vi "STAGE+mono+counter_edit11.vi"() -> ()   [LabVIEW 2017]
uses:
  Control 1.ctl
panel:
  out "XY Graph":cluster{dbl[], dbl[]}(graph)
  out "Slide":u8(slide) max=10 step=10 scale=0.0..10.0
  out "?":cluster{dbl[], "Y":T1}(graph)
  in  "?":enum32{"DELAY", "COUNTER", "MONO", "PLOT"}(tab)
  out "Final time [ps]":dbl
  out "Current time [ps]":dbl
  out "Initial time [ps]":dbl
  in  "Set this as t0":bool
  in  "Axis":i32=1
  in  "Motor ON":bool
  in  "Motor OFF":bool
  out "Current Position [mm]":dbl
  out "Final Position [mm]":dbl
  in  "Data Points":i32=100
  out "Current Point":i32
  in  "Step Size [um]":i32=10
  in  "Target [mm]":dbl format="%.3f"
  in  "Move":bool
  out "Initial position [mm]":dbl
  in  "GPIB address":string="23"
  in  "Count Mode":u16(ring) items=["A,B for Preset T", "A-B for Preset T", "A+B for Preset T", "A for Preset B"]
  in  "Trigger mode":u16(ring) items=["10 MHz"=0, "Input 2"=2, "Input T"=3]
  in  "Channel A Input":u16(ring)=1 items=["10 MHz", "Input 1"]
  in  "Channel B Input":u16(ring)=2 items=["Input 1"=1, "Input 2"=2]
  in  "Number of Measurements\n to take at one point/ Number of Periods":u16=1 min=1 max=2000 step=1
  in  "Time between measurements\n at one point (s)/Dwell Time":dbl=0.002 min=0.002 max=60.0 step=0.001
  in  "gate A mode (CW:0)":i16(slide) scale=0.0..2.0 scale format="%.2f"
  out "Counts":i32
  in  "Integrating time, 10^-7 sec":dbl=10000000.0
  out "Mono port":T2(ring)
  out "Time delay":u32=450000 min=1
  out "Serial":u32=12345
  in  "Step size":dbl=10.0 min=0.0
  in  "Scan to":i32=4000
  in  "Scan from":i32=2600
  out "Current wavelength":dbl
  out "Grt#":u8=1 min=1 max=3 step=1
  in  "?":bool
  out "Groove/mm":u32=1200
  out "Blaze (nm)":u32=300
  in  "Numeric 11":dbl
  in  "Numeric 10":dbl
  in  "Numeric 9":dbl
  in  "Numeric 8":dbl
  in  "Numeric 7":dbl
  in  "Numeric 6":dbl
  in  "Numeric 5":dbl
  in  "Numeric 4":dbl
  in  "Numeric 3":dbl
  in  "Numeric 2":dbl
  in  "Numeric":dbl
  out "Timeout 2":bool
  in  "?":bool
  out "Timeout":bool
  in  "Collect Data!":bool
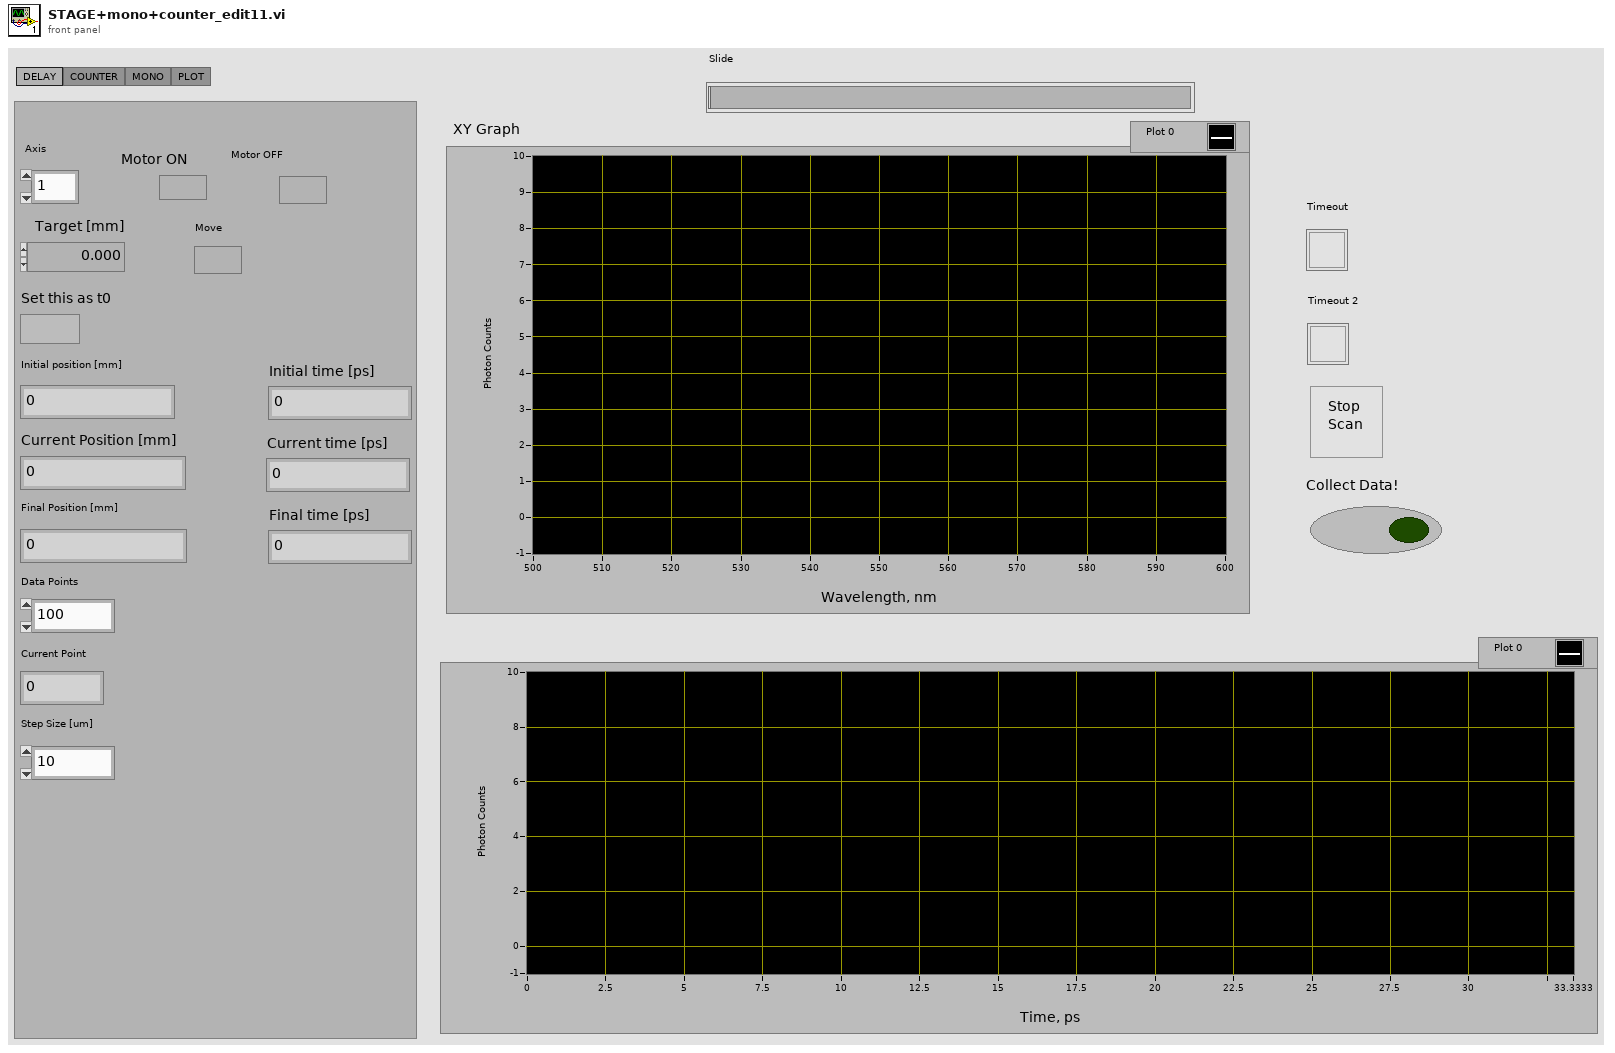
[diagram p1: front panel]
types:
  T1 = typedef "Control 1.ctl" = dbl[]
  T2 = enum8{"COM 1", "COM 2", "COM 3", "COM 4", "COM 5", "COM 6", "COM 7", "COM 8", "COM 9"}
  T3 = cluster{"input XON/XOFF":bool, "input HW Handshake":bool, "input alt HW HShk":bool, "output XON/XOFF":bool, "output HW Handshake":bool, "output alt HW HShk":bool, "XOFF byte":u8, "XON byte":u8, "parity error byte":u16}
  T4 = enum16{"no parity", "odd parity", "even parity", "mark parity", "space parity"}
  T5 = cluster{"Y[0]":dbl, "Y[1]":dbl, "Y[2]":dbl, "Y[3]":dbl, "Y[4]":dbl, "Y[5]":dbl, "Y[6]":dbl, "Y[7]":dbl, "Y[8]":dbl}
  T6 = typedef "NI_Matrix.lvlib/RealMatrix.ctl" = dbl[][]
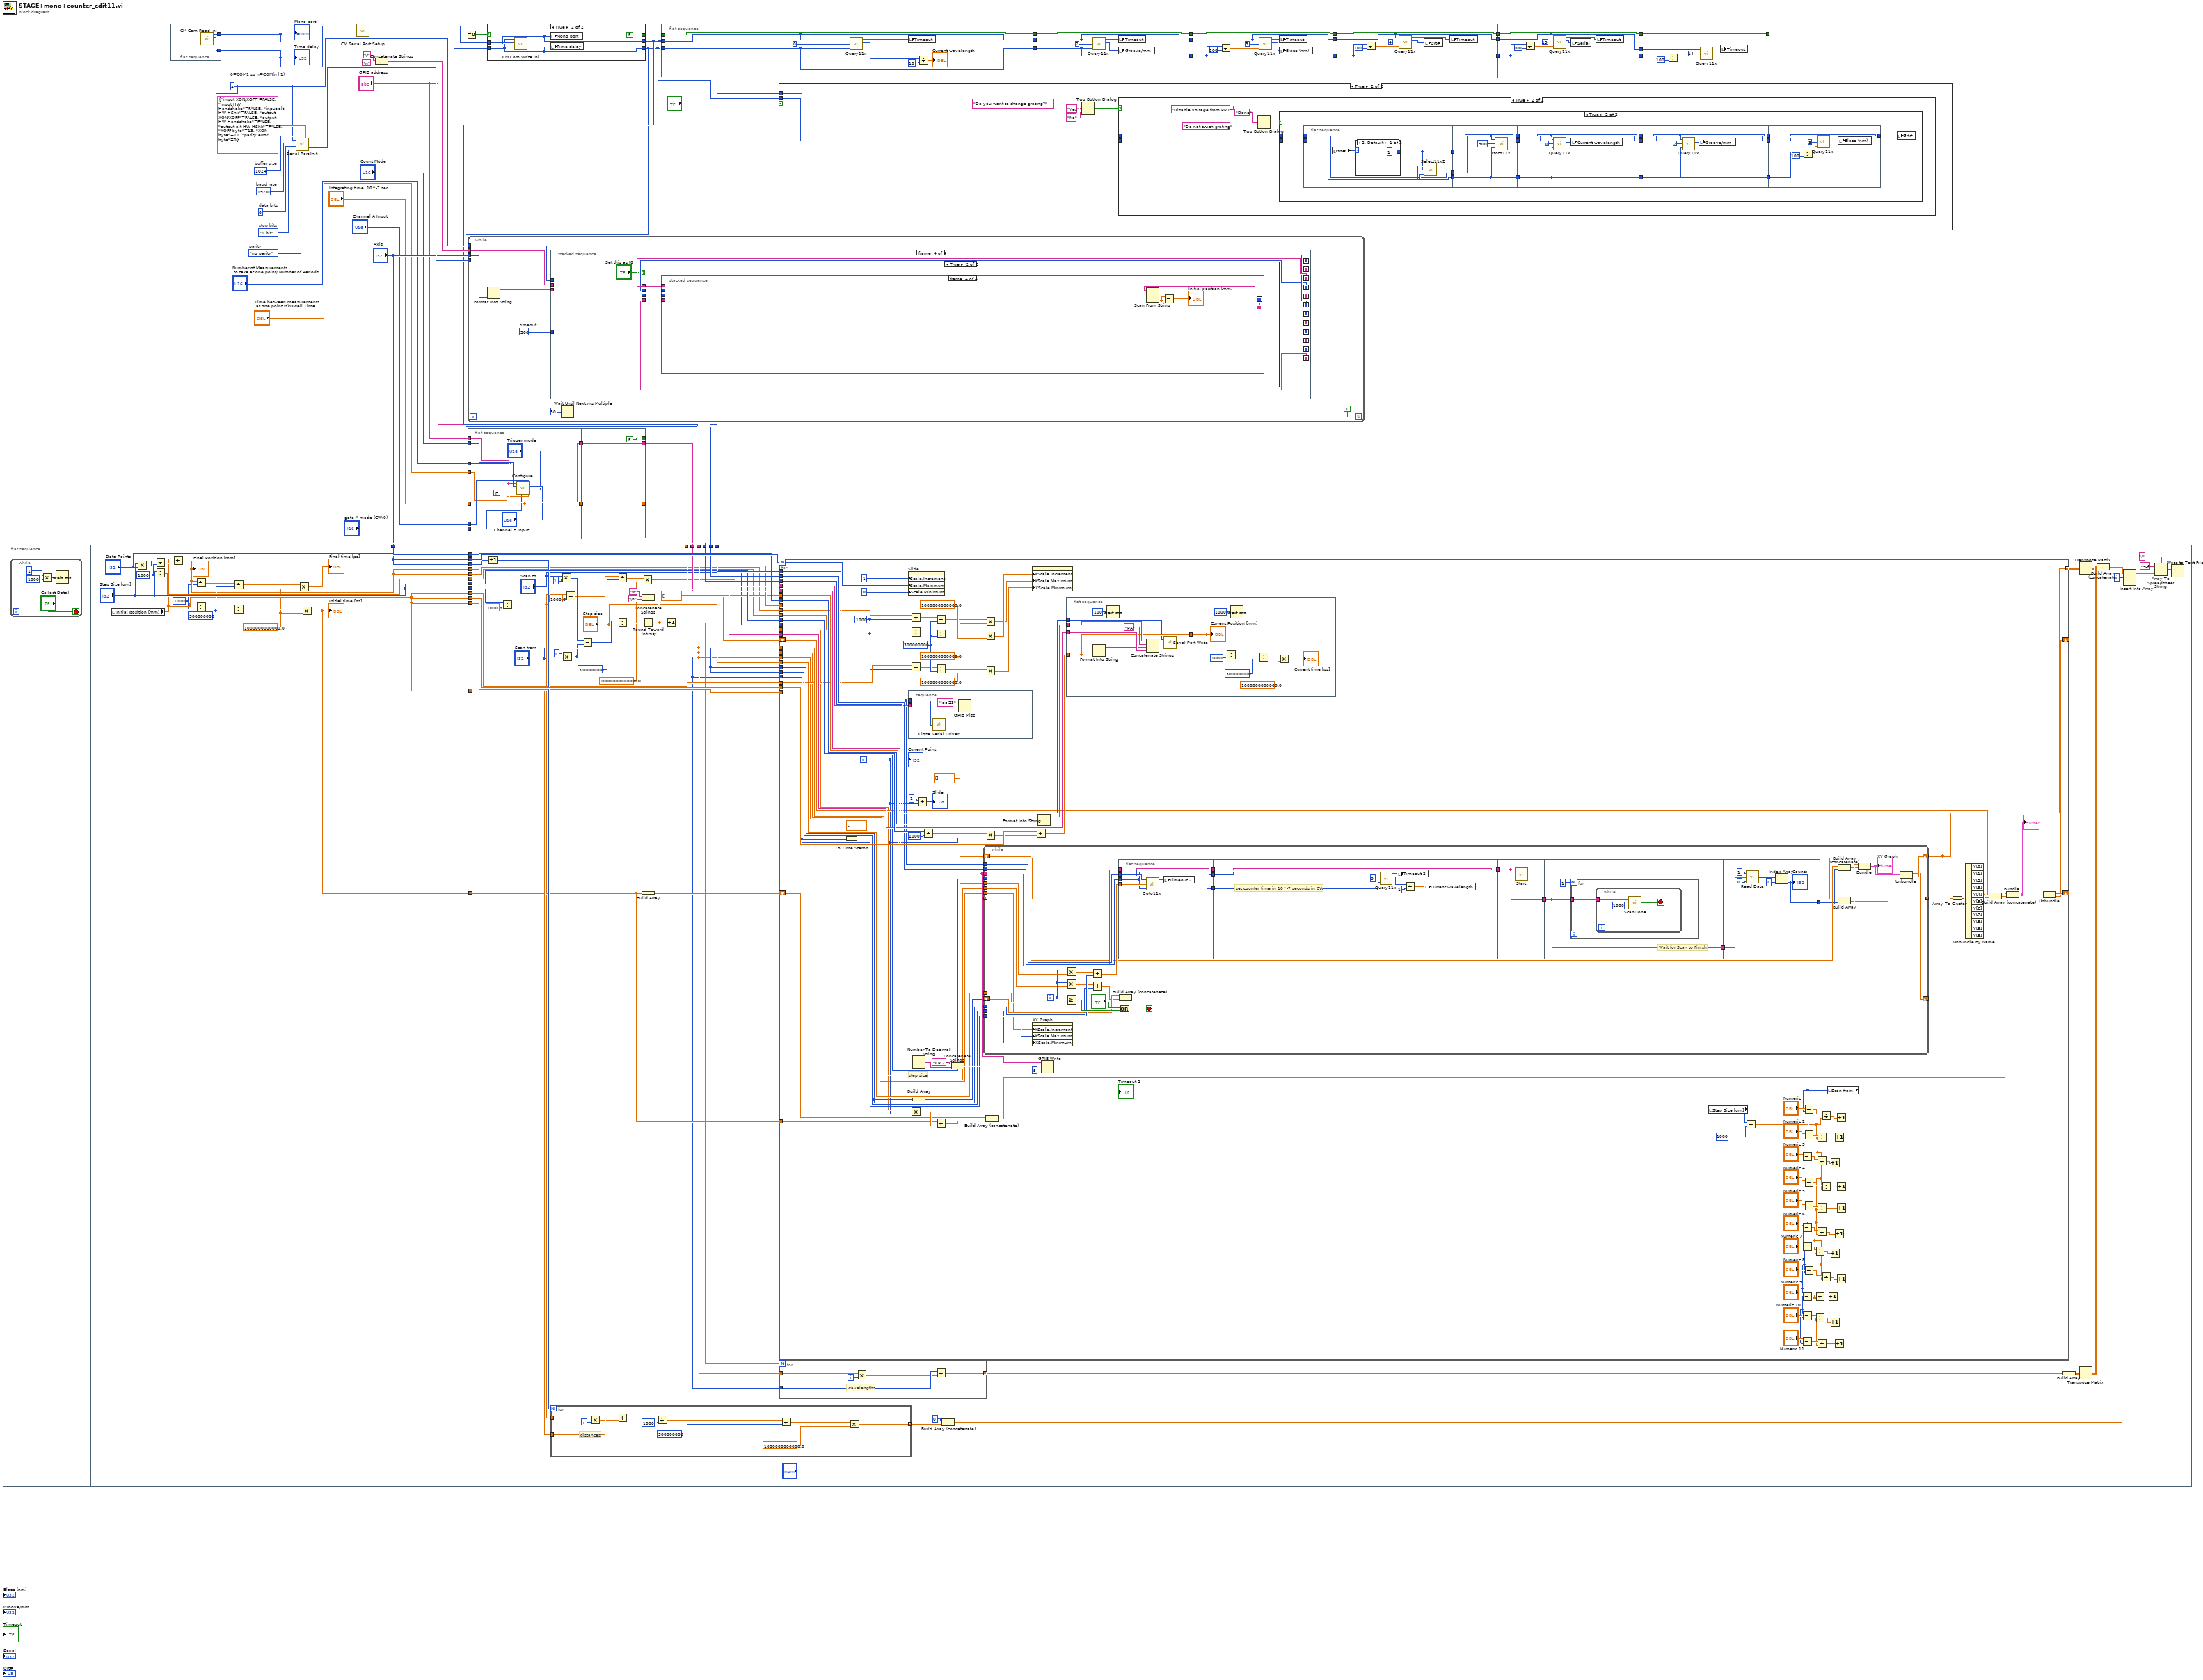
[diagram p0: block diagram]
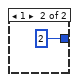
[diagram p5: hidden frame]
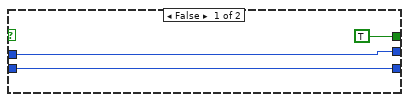
[diagram p6: hidden frame]
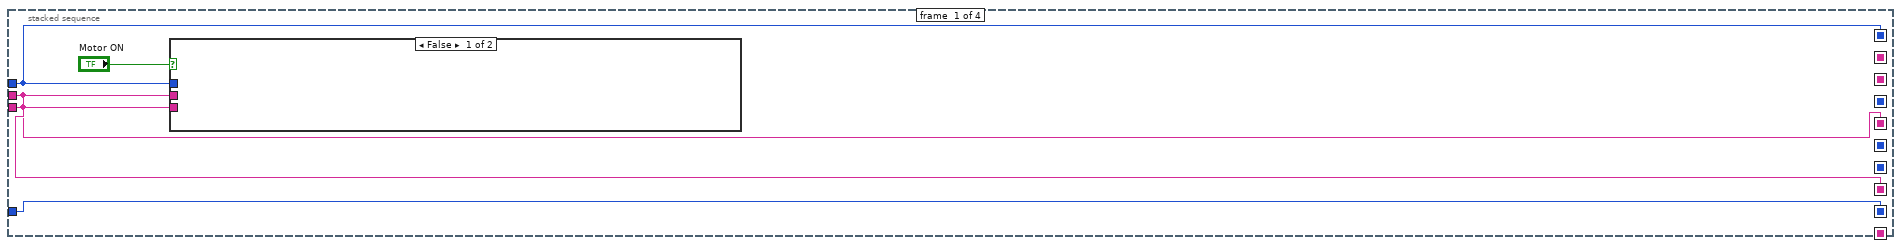
[diagram p7: hidden frame]
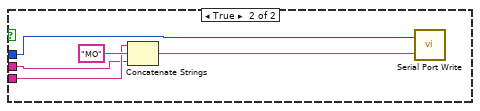
[diagram p8: hidden frame]
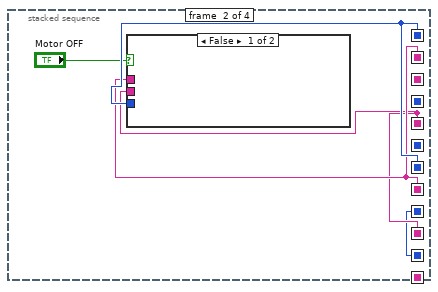
[diagram p9: hidden frame]
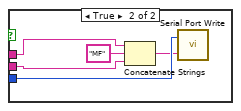
[diagram p10: hidden frame]
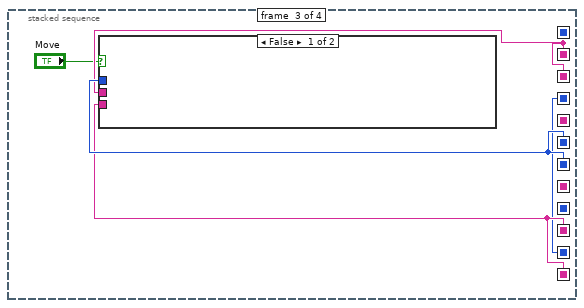
[diagram p11: hidden frame]
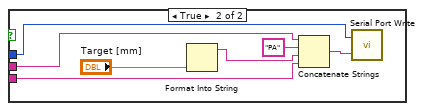
[diagram p12: hidden frame]
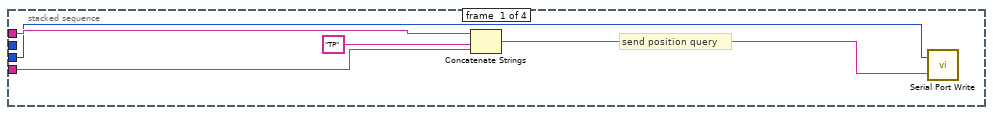
[diagram p14: hidden frame]
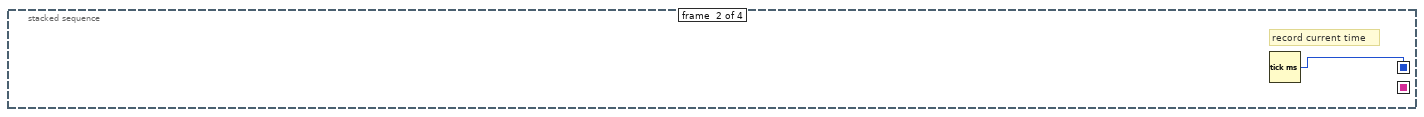
[diagram p15: hidden frame]
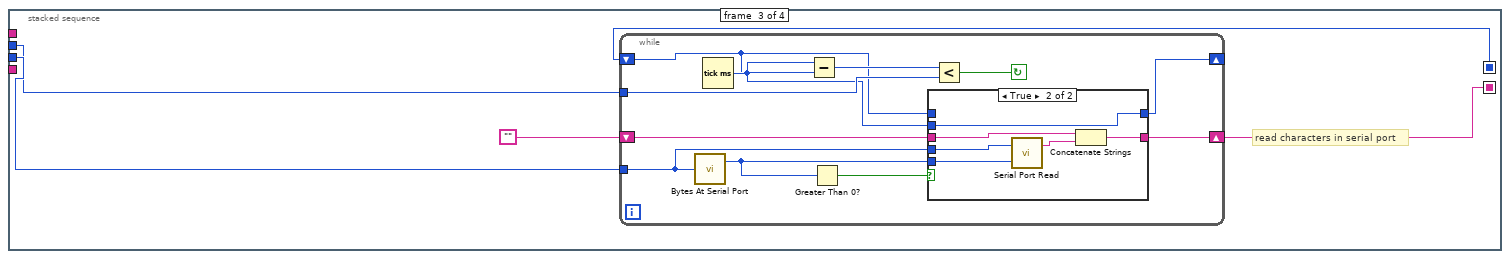
[diagram p16: hidden frame]
diagram:
  w55 = u32 19200  # baud rate
  w54 = u16 8  # data bits
  w53 = enum16{"1 bit", "1.5 bits", "2 bits"}."1 bit"  # stop bits
  w57 = T4."no parity"  # parity
  w52 = 4  # 0=COM1 so n=COM(n+1)
  w56 = u16 1024  # buffer size
  n1 = flat-sequence {
    tunnel: ["Data Points"] -> w61
    tunnel: "Axis" -> [w83]
    tunnel: [w75] -> w60
    tunnel: [w83] -> w59
    tunnel: ["Step Size [um]"] -> w12
    tunnel: [w75] -> w11
    tunnel: ["Step Size [um]"] -> w10
    tunnel: ["Data Points"] -> w9
    tunnel: [w75] -> w8
    tunnel: [w74] -> w7
    tunnel: [w75] -> w4
    tunnel: [w74] -> w3
    tunnel: [w77] -> w2
    tunnel: [w66] -> w1
    tunnel: w61 -> [w141]
    tunnel: w60 -> [w140]
    tunnel: w59 -> [w139]
    tunnel: w52 -> [w135]
    tunnel: w16 -> [w134]
    tunnel: w15 -> [w133]
    tunnel: w14 -> [w132]
    tunnel: "GPIB address" -> [w131]
    tunnel: w12 -> [w116]
    tunnel: w11 -> [w114]
    tunnel: w10 -> [w113]
    tunnel: w9 -> [w111]
    tunnel: w8 -> [w104]
    tunnel: w7 -> [w103]
    tunnel: w6 -> [w102]
    tunnel: w4 -> [w100]
    tunnel: w3 -> [w99]
    tunnel: w2 -> [w98]
    tunnel: w1 -> [w94]
    frame #0 {
      n2 = while {
        stop <- "Collect Data!" stop-if-true
        n3 = Multiply(x=1, y=1000) -> (x*y=w65:i32)
        n4 = Wait (ms)(milliseconds to wait=w65) -> ()  [unwired: 1 out]
      }
    }
    frame #1 {
      w67 = 1000000000000.0
      w73 = 1000
      w76 = 300000000
      w78 = 1000
      n5 = local read "Initial position [mm]"() -> (w75:dbl)
      n6 = Multiply(x="Step Size [um]", y="Data Points") -> (x*y=w82:i32)
      n7 = Divide(x=w82, y=w78) -> (x/y=w81:dbl)
      n8 = Divide(x="Step Size [um]", y=w78) -> (x/y=w77:dbl)
      n9 = Add(x=w75, y=w81) -> (x+y=w74:dbl)
      "Final Position [mm]" <- w74
      n10 = Divide(x=w74, y=w73) -> (x/y=w72:dbl)
      n11 = Divide(x=w75, y=w73) -> (x/y=w71:dbl)
      n12 = Divide(x=w72, y=w76) -> (x/y=w69:dbl)
      n13 = Divide(x=w71, y=w76) -> (x/y=w70:dbl)
      n14 = Multiply(x=w69, y=w67) -> (x*y=→"Final time [ps]":dbl)
      n15 = Multiply(x=w70, y=w67) -> (x*y=w66:dbl)
      "Initial time [ps]" <- w66
    }
    frame #2 {
      n16 = Increment(x=w111) -> (x+1=w112:i32)
      n17 = Divide(x=w116, y=1000.0) -> (x/y=w88:dbl)
      n18 = for {
        N: w112 -> [_]
        tunnel: w88 -> [w152]
        tunnel: w114 -> [w150]
        tunnel: [w143] -> w110 mode=indexing
        i -> [w151]
        # "distances"
        n19 = Multiply(x=w152, y=w151) -> (x*y=w149:dbl)
        n20 = Add(x=w150, y=w149) -> (x+y=w148:dbl)
        n21 = Divide(x=w148, y=1000) -> (x/y=w142:dbl)
        n22 = Divide(x=w142, y=300000000) -> (x/y=w145:dbl)
        n23 = Multiply(x=w145, y=1000000000000.0) -> (x*y=w143:dbl)
      }
      n24 = Multiply(x="Scan to", y=1) -> (x*y=w95:i32)
      n25 = Multiply(x=1, y="Scan from") -> (x*y=w84:i32)
      n26 = Divide(x=w88, y=1000.0) -> (x/y=w89:dbl)
      n27 = Subtract(x=w95, y=w84) -> (x-y=w126:i32)
      n28 = Divide(x=w89, y=300000000) -> (x/y=w91:dbl)
      n29 = Divide(x=w126, y="Step size") -> (x/y=w125:dbl)
      n30 = Multiply(x=w91, y=1000000000000.0) -> (x*y=w87:dbl)
      n31 = Concatenate Strings("\r", "\n") -> (w136:string)
      n32 = Round Toward -Infinity(1:w125) -> (0:w124:dbl)
      n33 = Build Array(w94) -> (w96:dbl[])
      n34 = Increment(x=w124) -> (x+1=w123:dbl)
      n35 = for {
        N: w141 -> [w226]
        tunnel: w140 -> [w262]
        tunnel: w113 -> [w258]
        tunnel: w139 -> [w255]
        tunnel: w136 -> [w252]
        tunnel: w135 -> [w253]
        tunnel: w134 -> [w251]
        tunnel: w133 -> [w248]
        tunnel: w132 -> [w250]
        tunnel: w131 -> [w249]
        tunnel: [w158] -> w119 mode=indexing
        tunnel: w84 -> [w243]
        tunnel: "Step size" -> [w242]
        tunnel: w124 -> [w241]
        tunnel: w104 -> [_]
        tunnel: w103 -> [_]
        tunnel: w102 -> [w239]
        tunnel: "Scan to" -> [w238]
        tunnel: "Scan from" -> [w237]
        tunnel: "Step size" -> [w197]
        tunnel: w100 -> [w221]
        tunnel: w99 -> [w219]
        tunnel: w98 -> [w222]
        tunnel: w87 -> [w206]
        shift-right: [w235] -> _
        shift-left: w96 -> [w200]
        shift-right: [w232] -> _
        shift-left: T1 [] ("Y") -> [w231]
        tunnel: w94 -> [w230]
        tunnel: "Scan from" -> [w198]
        tunnel: "Step size" -> [w199]
        i -> [w205]
        w220 = 1000
        w223 = 300000000
        # "step size"
        n36 = To Time Stamp(1:w243) -> ()  [unwired: 1 out]
        n37 = property on="Slide" class="Slide (strict)"("Scale.Increment"=1, "Scale.Maximum"=w226, "Scale.Minimum"=0) -> ()  [unwired: 2 in, 2 out]
        n38 = stacked-sequence {
          tunnel: w248 -> [w325]
          tunnel: w249 -> [_]
          frame #0 {
            n39 = call <vilib>:"Close Serial Driver.vi"("port number"=w325) -> ()  [unwired: 1 out]
            n40 = GPIB Misc(0:"loc 23" ("command string")) -> ()  [unwired: 1 in, 3 out]
          }
        }
        n41 = Divide(x=w219, y=w220) -> (x/y=w216:dbl)
        n42 = Divide(x=w222, y=w220) -> (x/y=w218:dbl)
        n43 = Divide(x=w221, y=w220) -> (x/y=w217:dbl)
        n44 = Multiply(x=w206, y=w205) -> (x*y=w236:dbl)
        n45 = Number To Decimal String(number=w239) -> (decimal integer string=w246:string)  [unwired: 1 in]
        n46 = Build Array(w198) -> (w202:i32[])
        n47 = Add(x=1, y=w205) -> (x+y=→"Slide":i32)
        n48 = Divide(x=w258, y=1000) -> (x/y=w257:dbl)
        n49 = Divide(x=w216, y=w223) -> (x/y=w208:dbl)
        n50 = Divide(x=w218, y=w223) -> (x/y=w212:dbl)
        n51 = Divide(x=w217, y=w223) -> (x/y=w210:dbl)
        n52 = Add(x=w230, y=w236) -> (x+y=w229:dbl)
        n53 = Concatenate Strings("CP 2,", w246) -> (w244:string)
        n54 = while {
          tunnel: w248 -> [w296]
          tunnel: w250 -> [w295]
          tunnel: w251 -> [w291]
          tunnel: w243 -> [w283]
          tunnel: w242 -> [w282]
          tunnel: w241 -> [w281]
          tunnel: w238 -> [w267]
          tunnel: w237 -> [w266]
          tunnel: w197 -> [w265]
          tunnel: w199 -> [w279]
          shift-right: [w274] -> w158
          shift-left: dbl[] [] ("Y") -> [w272]
          shift-right: [w273] -> _
          shift-left: w202 -> [w277]
          tunnel: w198 -> [w270]
          tunnel: dbl[] [] ("Y") -> [w263] mode=indexing
          tunnel: [w264] -> _ mode=indexing
          i -> [w280]
          stop <- w294 stop-if-true
          n55 = property on="XY Graph" class="XYGraph (strict)"("XScale.Increment"=w265, "XScale.Maximum"=w267, "XScale.Minimum"=w266) -> ()  [unwired: 2 in, 2 out]
          n56 = Multiply(x=w280, y=w282) -> (x*y=w297:dbl)
          n57 = Multiply(x=w280, y=w279) -> (x*y=w278:dbl)
          n58 = Greater Or Equal?(x=w280, y=w281) -> (x >= y?=w292:bool)
          n59 = Add(x=w297, y=w283) -> (x+y=w284:dbl)
          n60 = Add(x=w278, y=w270) -> (x+y=w276:dbl)
          n61 = flat-sequence {
            tunnel: w284 -> [w302]
            tunnel: w296 -> [w301]
            tunnel: [w301] -> w290
            tunnel: w295 -> [w300]
            tunnel: [w300] -> w289
            tunnel: w291 -> [w298]
            tunnel: [w298] -> w288
            tunnel: w290 -> [w309]
            tunnel: w289 -> [w308]
            tunnel: w288 -> [w306]
            tunnel: [w306] -> w287
            tunnel: w287 -> [w311]
            tunnel: [w311] -> w286
            tunnel: w286 -> [w312]
            tunnel: [w312] -> w285
            tunnel: w285 -> [w319]
            tunnel: [w318] -> w269
            frame #0 {
              n62 = call "Goto11x.vi"("time delay"=w300, "WAVELENGTH"=w302, "port number"=w301) -> ("timeout"=w299:bool)  [unwired: 2 out]
              n63 = local write "Timeout 2"(w299) -> ()
            }
            frame #1 {
              # "set counter time in 10^-7 seconds in CW"
              n64 = call "Query11x.vi"("port number"=w309, "QUERY"=0, "time delay"=w308) -> ("timeout"=w307:bool, "STATUS MESSAGE"=w305:u16)  [unwired: 2 out]
              n65 = local write "Timeout 2"(w307) -> ()
              n66 = Divide(x=w305, y=1) -> (x/y=w304:dbl)
              n67 = local write "Current wavelength"(w304) -> ()
            }
            frame #2 {
              n68 = call "Start.vi"("GPIB Address"=w311) -> ()  [unwired: 9 in]
            }
            frame #3 {
              # "Wait for Scan to Finish"
              n69 = for {
                N: 1 -> [_]
                tunnel: w312 -> [w314]
                n70 = while {
                  tunnel: w314 -> [w315]
                  stop <- w317 stop-if-true
                  n71 = call "ScanDone.vi"("Wait (ms)"=1000, "GPIB Address"=w315) -> ("Scan Finished?"=w317:bool)
                }
              }
            }
            frame #4 {
              n72 = call "Read Data.vi"("Channel Number"=0, "GPIB Address"=w319, "Number of Datapoints"=1) -> ("Data"=w320:i32[])
              n73 = Index Array(array=w320, index=0) -> (element=w318:i32)
              "Counts" <- w318
            }
          }
          n74 = Or(x="?", y=w292) -> (x .or. y?=w294:bool)
          n75 = Build Array (concatenate)(w277, w276) -> (w275:dbl[])
          n76 = Build Array (concatenate)(w272, w269) -> (w271:dbl[])
          n77 = Build Array(w263, w269) -> (w264:dbl[])
          n78 = Bundle(w275, w271) -> (w268:cluster{dbl[], dbl[]})  [unwired: 1 in]
          "XY Graph" <- w268
          n79 = Unbundle(w268) -> (w273:dbl[], w274:dbl[])
        }
        n80 = Multiply(x=w208, y=1000000000000.0) -> (x*y=w207:dbl)
        n81 = Multiply(x=w212, y=1000000000000.0) -> (x*y=w211:dbl)
        n82 = Multiply(x=w210, y=1000000000000.0) -> (x*y=w209:dbl)
        n83 = Multiply(x=w257, y=w205) -> (x*y=w261:dbl)
        n84 = Build Array (concatenate)(w200, w229) -> (w228:dbl[])
        n85 = property class="XYGraph (strict)"("XScale.Increment"=w211, "XScale.Maximum"=w207, "XScale.Minimum"=w209) -> ()  [unwired: 2 in, 2 out]
        n86 = Add(x=w262, y=w261) -> (x+y=w260:dbl)
        n87 = Format Into String(w255) -> (resulting string=w254:string)  [unwired: 3 in, 1 out]
        n88 = GPIB Write(0:w251, 1:w244, 2:i16 5 ("mode (0)")) -> ()  [unwired: 2 in, 2 out]
        n89 = flat-sequence {
          tunnel: w260 -> [w328]
          tunnel: [w328] -> w256
          tunnel: w252 -> [w330]
          tunnel: w254 -> [w329]
          tunnel: w253 -> [w326]
          tunnel: w256 -> [w339]
          frame #0 {
            n90 = Format Into String(w328) -> (resulting string=w327:string)  [unwired: 3 in, 1 out]
            n91 = Wait (ms)(milliseconds to wait=u32 100) -> ()  [unwired: 1 out]
            n92 = Concatenate Strings(w329, "PA" ("Substring"), w327, w330) -> (w332:string)
            n93 = call <vilib>:"Serial Port Write.vi"("string to write"=w332, "port number"=w326) -> ()  [unwired: 1 out]
          }
          frame #1 {
            n94 = Divide(x=w339, y=1000) -> (x/y=w337:dbl)
            n95 = Wait (ms)(milliseconds to wait=u32 1000) -> ()  [unwired: 1 out]
            n96 = Divide(x=w337, y=300000000) -> (x/y=w336:dbl)
            n97 = Multiply(x=w336, y=1000000000000.0) -> (x*y=→"Current time [ps]":dbl)
            "Current Position [mm]" <- w339
          }
        }
        n98 = local read "Step Size [um]"() -> (w173:i32)
        n99 = Divide(x=w173, y=1000) -> (x/y=w171:dbl)
        n100 = local read "Scan from"() -> (w185:i32)
        n101 = Subtract(x="Numeric 3", y=w185) -> (x-y=w182:dbl)
        n102 = Subtract(x="Numeric 6", y=w185) -> (x-y=w179:dbl)
        n103 = Subtract(x="Numeric 7", y=w185) -> (x-y=w178:dbl)
        n104 = Subtract(x="Numeric 9", y=w185) -> (x-y=w176:dbl)
        n105 = Subtract(x="Numeric 10", y=w185) -> (x-y=w175:dbl)
        n106 = Subtract(x="Numeric 11", y=w185) -> (x-y=w174:dbl)
        n107 = Subtract(x="Numeric", y=w185) -> (x-y=w184:dbl)
        n108 = Subtract(x="Numeric 2", y=w185) -> (x-y=w183:dbl)
        n109 = Subtract(x="Numeric 4", y=w185) -> (x-y=w181:dbl)
        n110 = Subtract(x="Numeric 5", y=w185) -> (x-y=w180:dbl)
        n111 = Subtract(x="Numeric 8", y=w185) -> (x-y=w177:dbl)
        n112 = Divide(x=w178, y=w171) -> (x/y=w164:dbl)
        n113 = Divide(x=w176, y=w171) -> (x/y=w162:dbl)
        n114 = Divide(x=w175, y=w171) -> (x/y=w161:dbl)
        n115 = Divide(x=w183, y=w171) -> (x/y=w169:dbl)
        n116 = Divide(x=w182, y=w171) -> (x/y=w168:dbl)
        n117 = Divide(x=w180, y=w171) -> (x/y=w166:dbl)
        n118 = Divide(x=w179, y=w171) -> (x/y=w165:dbl)
        n119 = Divide(x=w174, y=w171) -> (x/y=w160:dbl)
        n120 = Divide(x=w184, y=w171) -> (x/y=w170:dbl)
        n121 = Divide(x=w181, y=w171) -> (x/y=w167:dbl)
        n122 = Divide(x=w177, y=w171) -> (x/y=w163:dbl)
        n123 = Increment(x=w162) -> ()  [unwired: 1 out]
        n124 = Increment(x=w168) -> ()  [unwired: 1 out]
        n125 = Increment(x=w164) -> ()  [unwired: 1 out]
        n126 = Increment(x=w161) -> ()  [unwired: 1 out]
        n127 = Increment(x=w169) -> ()  [unwired: 1 out]
        n128 = Increment(x=w165) -> ()  [unwired: 1 out]
        n129 = Increment(x=w160) -> ()  [unwired: 1 out]
        n130 = Increment(x=w170) -> ()  [unwired: 1 out]
        n131 = Increment(x=w167) -> ()  [unwired: 1 out]
        n132 = Increment(x=w166) -> ()  [unwired: 1 out]
        n133 = Increment(x=w163) -> ()  [unwired: 1 out]
        n134 = Array To Cluster(array=w158) -> (cluster=w240:T5)
        n135 = Unbundle By Name(w240) -> ("Y[4]"=w234:dbl)  [unwired: 10 out]
        n136 = Build Array (concatenate)(w231, w234) -> (w233:T1)
        n137 = Bundle(w228, "Y"=w233) -> (w227:cluster{dbl[], "Y":T1})  [unwired: 1 in]
        "?" <- w227
        n138 = Unbundle(w227) -> (w235:dbl[], "Y"=w232:T1)
        "Current Point" <- w205
      }
      n139 = for {
        N: w123 -> [_]
        tunnel: "Step size" -> [w157]
        tunnel: w84 -> [w155]
        tunnel: [w153] -> w121 mode=indexing
        i -> [w156]
        # "wavelengths"
        n140 = Multiply(x=w157, y=w156) -> (x*y=w154:dbl)
        n141 = Add(x=w155, y=w154) -> (x+y=w153:dbl)
      }
      n142 = Build Array (concatenate)(0, w110) -> (w107:dbl[])
      n143 = Build Array(w121) -> (w120:dbl[][])
      n144 = Transpose Matrix(1:w119) -> (0:w117:dbl[][])
      n145 = Transpose Matrix(1:w120) -> (0:w118:dbl[][])
      n146 = Build Array (concatenate)(w118, w117) -> (w106:T6)
      n147 = Insert Into Array(array=w106, index (row)=0, new element=w107) -> (w105:T6)  [unwired: 1 in]
      n148 = Array To Spreadsheet String(delimiter (Tab)=",", array=w105, 3:"%f" ("format string")) -> (spreadsheet string=w122:string)
      n149 = Write to Text File(text=w122) -> ()  [unwired: 3 in, 3 out]
    }
  }
  n150 = flat-sequence {
    tunnel: [w343] -> w30
    tunnel: [w342] -> w29
    frame #0 {
      n151 = call "CM Com Read ini.vi"() -> ("Mono port"=w342:T2, "time delay1"=w343:u32)  [unwired: 7 in]
    }
  }
  n152 = call <vilib>:"Serial Port Init.vi"("flow control etc."=T3 {"input XON/XOFF"=FALSE, "input HW Handshake"=FALSE, "input alt HW HShk"=FALSE, "output XON/XOFF"=FALSE, "output HW Handshake"=FALSE, "output alt HW HShk"=FALSE, "XOFF byte"=13, "XON byte"=11, "parity error byte"=0}, "parity"=w57, "buffer size"=w56, "stop bits"=w53, "data bits"=w54, "baud rate"=w55, "port number"=w52) -> ("error code"=w51:i32)
  n153 = call "CM Serial Port Setup.vi"("COM port"=w29, "time delay"=w30) -> ("time delay1"=w25:u32, "DK port Out"=w26:T2, "error code"=w28:i32)  [unwired: 7 in]
  n154 = Concatenate Strings("\r", "\n") -> (w47:string)
  n155 = Equal To 0?(x=w28) -> (x = 0?=w27:bool)
  n156 = while {
    tunnel: w52 -> [w346]
    tunnel: w47 -> [w347]
    tunnel: w51 -> [_]
    tunnel: "Axis" -> [w344]
    stop <- TRUE continue-if-true
    w345 = u32 200  # timeout
    n157 = Format Into String(w344) -> (resulting string=w348:string)  [unwired: 3 in, 1 out]
    n158 = stacked-sequence {
      seq-local: [w353 _ _ _] -> [_ w364 _ _]
      seq-local: [w352 _ _ _] -> [_ w363 _ _]
      seq-local: [w354 _ _ _] -> [_ w365 _ _]
      seq-local: [w351 _ _ _] -> [_ w361 _ _]
      seq-local: [_ w364 _ _] -> [_ _ w374 _]
      seq-local: [_ w363 _ _] -> [_ _ w373 _]
      seq-local: [_ w365 _ _] -> [_ _ w375 _]
      seq-local: [_ w361 _ _] -> [_ _ w371 _]
      seq-local: [_ _ w374 _] -> [_ _ _ w387]
      seq-local: [_ _ w373 _] -> [_ _ _ w384]
      seq-local: [_ _ w375 _] -> [_ _ _ w386]
      seq-local: [_ _ w371 _] -> [_ _ _ w385]
      tunnel: w348 -> [w353 _ _ _]
      tunnel: w347 -> [w352 _ _ _]
      tunnel: w346 -> [w354 _ _ _]
      tunnel: w345 -> [w351 _ _ _]
      frame #0 {
        n159 = case shown="False" "Motor ON" {
          tunnel: w354 -> [_ w360]
          tunnel: w353 -> [_ w357]
          tunnel: w352 -> [_ w356]
          frame False {
          }
          frame True {
            n160 = Concatenate Strings(w357, "MO" ("Substring"), w356) -> (w358:string)
            n161 = call <vilib>:"Serial Port Write.vi"("string to write"=w358, "port number"=w360) -> ()  [unwired: 1 out]
          }
        }
      }
      frame #1 {
        n162 = case shown="False" "Motor OFF" {
          tunnel: w365 -> [_ w370]
          tunnel: w364 -> [_ w367]
          tunnel: w363 -> [_ w366]
          frame False {
          }
          frame True {
            n163 = Concatenate Strings(w367, "MF" ("Substring"), w366) -> (w368:string)
            n164 = call <vilib>:"Serial Port Write.vi"("string to write"=w368, "port number"=w370) -> ()  [unwired: 1 out]
          }
        }
      }
      frame #2 {
        n165 = case shown="False" "Move" {
          tunnel: w375 -> [_ w382]
          tunnel: w374 -> [_ w379]
          tunnel: w373 -> [_ w378]
          frame False {
          }
          frame True {
            n166 = Format Into String("Target [mm]") -> (resulting string=w376:string)  [unwired: 3 in, 1 out]
            n167 = Concatenate Strings(w379, "PA" ("Substring"), w376, w378) -> (w380:string)
            n168 = call <vilib>:"Serial Port Write.vi"("string to write"=w380, "port number"=w382) -> ()  [unwired: 1 out]
          }
        }
      }
      frame #3 {
        n169 = case shown="True" "Set this as t0" {
          tunnel: w387 -> [_ w391]
          tunnel: w386 -> [_ w390]
          tunnel: w385 -> [_ w389]
          tunnel: w384 -> [_ w388]
          frame False {
          }
          frame True {
            n170 = stacked-sequence {
              seq-local: [_ w397 _ _] -> [_ _ w399 _]
              seq-local: [_ _ w398 _] -> [_ _ _ w424]
              tunnel: w391 -> [w394 _ _ _]
              tunnel: w390 -> [w393 _ w402 _]
              tunnel: w389 -> [_ _ w400 _]
              tunnel: w388 -> [w392 _ _ _]
              frame #0 {
                # "send position query"
                n171 = Concatenate Strings(w394, "TP" ("Substring"), w392) -> (w395:string)
                n172 = call <vilib>:"Serial Port Write.vi"("string to write"=w395, "port number"=w393) -> ()  [unwired: 1 out]
              }
              frame #1 {
                # "record current time"
                n173 = Tick Count (ms)() -> (millisecond timer value=w397:u32)
              }
              frame #2 {
                # "read characters in serial port"
                n174 = while {
                  shift-left: w399 -> [w403]
                  shift-right: [w404] -> _
                  tunnel: w400 -> [w407]
                  shift-left: "" -> [w410]
                  shift-right: [w409] -> w398
                  tunnel: w402 -> [w411]
                  stop <- w406 continue-if-true
                  n175 = call <vilib>:"Bytes At Serial Port.vi"("port number"=w411) -> ("byte count"=w412:u32)  [unwired: 1 out]
                  n176 = Tick Count (ms)() -> (millisecond timer value=w405:u32)
                  n177 = Subtract(x=w405, y=w403) -> (x-y=w408:u32)
                  n178 = Greater Than 0?(x=w412) -> (x > 0?=w413:bool)
                  n179 = case shown="True" w413 {
                    tunnel: w412 -> [_ w421]
                    tunnel: w411 -> [_ w420]
                    tunnel: w410 -> [w415 w418]
                    tunnel: [w415 w417] -> w409
                    tunnel: [w414 w416] -> w404
                    tunnel: w405 -> [_ w416]
                    tunnel: w403 -> [w414 _]
                    frame False {
                    }
                    frame True {
                      n180 = call <vilib>:"Serial Port Read.vi"("requested byte count"=w421, "port number"=w420) -> ("string read"=w419:string)  [unwired: 1 out]
                      n181 = Concatenate Strings(w418, w419) -> (w417:string)
                    }
                  }
                  n182 = Less?(x=w408, y=w407) -> (x < y?=w406:bool)
                }
              }
              frame #3 {
                n183 = Scan From String(input string=w424) -> (output 1=w422:dbl)  [unwired: 4 in, 3 out]
                n184 = Subtract(x=w422, y=w422) -> (x-y=→"Initial position [mm]":dbl)
              }
            }
          }
        }
      }
    }
    n185 = Wait Until Next ms Multiple(millisecond multiple=u32 50) -> ()  [unwired: 1 out]
  }
  n186 = flat-sequence {
    tunnel: "GPIB address" -> [w432]
    tunnel: [w432] -> w31
    tunnel: "Count Mode" -> [w433]
    tunnel: "Number of Measurements\n to take at one point/ Number of Periods" -> [w430]
    tunnel: "Time between measurements\n at one point (s)/Dwell Time" -> [w429]
    tunnel: "Channel A Input" -> [w434]
    tunnel: "gate A mode (CW:0)" -> [w426]
    tunnel: "Integrating time, 10^-7 sec" -> [w425]
    tunnel: [w425] -> w5
    tunnel: w31 -> [w436]
    tunnel: [w436] -> w16
    tunnel: [FALSE] -> _
    tunnel: [w435] -> w6
    tunnel: w5 -> [w435]
    frame #0 {
      n187 = call "Configure.vi"("Dwell Time (s)"=w429, "Channel T Input"="Trigger mode", "Channel B Input"="Channel B Input", "Channel A Input"=w434, "Integrating time, 10^-7 sec"=w425, "gate mode (CW:0)"=w426, "Scan End Mode"=FALSE, "Number of Periods"=w430, "Count Mode"=w433, "GPIB Address"=w432) -> ()
    }
    frame #1 {
    }
  }
  n188 = case shown="True" w27 {
    tunnel: w26 -> [w440 w443]
    tunnel: w25 -> [w439 w442]
    tunnel: [w440 w443] -> w15
    tunnel: [w439 w442] -> w14
    tunnel: [TRUE FALSE] -> w24
    frame False {
    }
    frame True {
      n189 = call "CM Com Write ini.vi"("time delay1"=w443, "Mono port"=w442) -> ()  [unwired: 7 in]
      n190 = local write "Mono port"(w443) -> ()
      n191 = local write "Time delay"(w442) -> ()
    }
  }
  n192 = flat-sequence {
    tunnel: w14 -> [w449]
    tunnel: [w449] -> w46
    tunnel: w15 -> [w451]
    tunnel: [w451] -> w45
    tunnel: w24 -> [w447]
    tunnel: [w447] -> w44
    tunnel: w46 -> [w454]
    tunnel: [w454] -> w43
    tunnel: w45 -> [w456]
    tunnel: [w456] -> w42
    tunnel: w44 -> [w452]
    tunnel: [w452] -> w41
    tunnel: w43 -> [w464]
    tunnel: [w464] -> w40
    tunnel: w42 -> [w461]
    tunnel: [w461] -> w39
    tunnel: w41 -> [w458]
    tunnel: [w458] -> w38
    tunnel: w40 -> [w472]
    tunnel: [w472] -> w37
    tunnel: w39 -> [w469]
    tunnel: [w469] -> w36
    tunnel: w38 -> [w466]
    tunnel: [w466] -> w35
    tunnel: w37 -> [w480]
    tunnel: [w480] -> w34
    tunnel: w36 -> [w477]
    tunnel: [w477] -> w33
    tunnel: w35 -> [w474]
    tunnel: [w474] -> w32
    tunnel: w34 -> [w487]
    tunnel: w33 -> [w484]
    tunnel: [w482] -> _
    tunnel: w32 -> [w482]
    frame #0 {
      n193 = call "Query11x.vi"("port number"=w451, "QUERY"=u16 0, "time delay"=w449) -> ("timeout"=w448:bool, "STATUS MESSAGE"=w446:u16)  [unwired: 2 out]
      n194 = local write "Timeout"(w448) -> ()
      n195 = Divide(x=w446, y=10 ("Numeric")) -> (x/y=→"Current wavelength":dbl)
    }
    frame #1 {
      n196 = call "Query11x.vi"("port number"=w456, "QUERY"=u16 2, "time delay"=w454) -> ("timeout"=w453:bool, "STATUS MESSAGE"=w455:u16)  [unwired: 2 out]
      n197 = local write "Timeout"(w453) -> ()
      n198 = local write "Groove/mm"(w455) -> ()
    }
    frame #2 {
      n199 = Divide(x=w464, y=i16 100 ("device (1)")) -> (x/y=w462:dbl)
      n200 = call "Query11x.vi"("port number"=w461, "QUERY"=u16 3, "time delay"=w462) -> ("timeout"=w459:bool, "STATUS MESSAGE"=w460:u16)  [unwired: 2 out]
      n201 = local write "Timeout"(w459) -> ()
      n202 = local write "Blaze (nm)"(w460) -> ()
    }
    frame #3 {
      n203 = Divide(x=w472, y=i16 100 ("device (1)")) -> (x/y=w470:dbl)
      n204 = call "Query11x.vi"("port number"=w469, "QUERY"=u16 4, "time delay"=w470) -> ("timeout"=w467:bool, "STATUS MESSAGE"=w468:u16)  [unwired: 2 out]
      n205 = local write "Grt#"(w468) -> ()
      n206 = local write "Timeout"(w467) -> ()
    }
    frame #4 {
      n207 = Divide(x=w480, y=i16 100 ("device (1)")) -> (x/y=w478:dbl)
      n208 = call "Query11x.vi"("port number"=w477, "QUERY"=u16 19, "time delay"=w478) -> ("timeout"=w475:bool, "STATUS MESSAGE"=w476:u16)  [unwired: 2 out]
      n209 = local write "Serial"(w476) -> ()
      n210 = local write "Timeout"(w475) -> ()
    }
    frame #5 {
      n211 = Divide(x=w487, y=i16 100 ("device (1)")) -> (x/y=w485:dbl)
      n212 = call "Query11x.vi"("port number"=w484, "QUERY"=u16 14, "time delay"=w485) -> ("timeout"=w483:bool)  [unwired: 3 out]
      n213 = local write "Timeout"(w483) -> ()
    }
  }
  n214 = case shown="True" "?" {
    tunnel: w14 -> [_ w490]
    tunnel: w15 -> [_ w489]
    frame False {
    }
    frame True {
      n215 = Two Button Dialog(message="Do you want to change grating?", 1:"No" ("F button name (\"Cancel\")"), 2:"Yes" ("T button name (\"OK\")")) -> (T button?=w491:bool)
      n216 = case shown="True" w491 {
        tunnel: w490 -> [_ w496]
        tunnel: w489 -> [_ w495]
        frame False {
        }
        frame True {
          n217 = Two Button Dialog(message="Disable voltage from PMT", 1:"Do not swich grating" ("F button name (\"Cancel\")"), 2:"Done" ("T button name (\"OK\")")) -> (T button?=w497:bool)
          n218 = case shown="True" w497 {
            tunnel: w496 -> [_ w515]
            tunnel: w495 -> [_ w514]
            frame False {
            }
            frame True {
              n219 = flat-sequence {
                tunnel: w515 -> [w519]
                tunnel: [w519] -> w512
                tunnel: w514 -> [w518]
                tunnel: [w518] -> w511
                tunnel: [w516] -> w510
                tunnel: w512 -> [w523]
                tunnel: [w523] -> w509
                tunnel: w511 -> [w524]
                tunnel: [w524] -> w508
                tunnel: w510 -> [w522]
                tunnel: [w522] -> w507
                tunnel: w509 -> [w530]
                tunnel: [w530] -> w506
                tunnel: w508 -> [w529]
                tunnel: [w529] -> w505
                tunnel: w507 -> [w527]
                tunnel: [w527] -> w504
                tunnel: w506 -> [w533]
                tunnel: [w533] -> w503
                tunnel: w505 -> [w534]
                tunnel: [w534] -> w502
                tunnel: w504 -> [w531]
                tunnel: [w531] -> w501
                tunnel: w503 -> [w538]
                tunnel: w502 -> [w539]
                tunnel: [w536] -> w513
                tunnel: w501 -> [w536]
                frame #0 {
                  n220 = local read "Grt#"() -> (w517:u8)
                  n221 = case shown="2, Default" w517 {
                    tunnel: [1 2] -> w516
                    frame 2, Default {
                    }
                    frame 1 {
                    }
                  }
                  n222 = call "Select11x2.vi"("time delay"=w519, "NEW GRT?"=w516, "port number"=w518) -> ()  [unwired: 3 out]
                }
                frame #1 {
                  n223 = call "Goto11x.vi"("time delay"=w523, "WAVELENGTH"=u16 300, "port number"=w524) -> ()  [unwired: 3 out]
                }
                frame #2 {
                  n224 = call "Query11x.vi"("port number"=w529, "QUERY"=u16 0, "time delay"=w530) -> ("STATUS MESSAGE"=w526:u16)  [unwired: 3 out]
                  n225 = local write "Current wavelength"(w526) -> ()
                }
                frame #3 {
                  n226 = call "Query11x.vi"("port number"=w534, "QUERY"=u16 2, "time delay"=w533) -> ("STATUS MESSAGE"=w532:u16)  [unwired: 3 out]
                  n227 = local write "Groove/mm"(w532) -> ()
                }
                frame #4 {
                  n228 = Divide(x=w538, y=i16 100 ("device (1)")) -> (x/y=w540:dbl)
                  n229 = call "Query11x.vi"("port number"=w539, "QUERY"=u16 3, "time delay"=w540) -> ("STATUS MESSAGE"=w537:u16)  [unwired: 3 out]
                  n230 = local write "Blaze (nm)"(w537) -> ()
                }
              }
              n231 = local write "Grt#"(w513) -> ()
            }
          }
        }
      }
    }
  }
  "Mono port" <- w29
  "Time delay" <- w30
